vi "Create Multiline String Picture.vi"(11 "array of strings":string[](array[string])) -> (3 "string picture":picture)   [LabVIEW 2017]
doc: "Converts each string from <b>array of strings</b> into picture using custom font (Default Settings.vi:font) and places one under the other in the <b>string picture</b>."
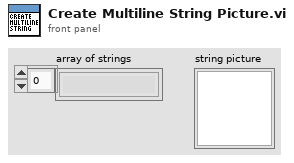
[diagram p1: front panel]
types:
  T1 = typedef "imagedata.ctl" = cluster{"image type":i32, "image depth":i32, "image":u8[], "mask":u8[], "colors":u32[], "Rectangle":cluster{"left":i16, "top":i16, "right":i16, "bottom":i16}}
  T2 = cluster{"left":i16, "top":i16, "right":i16, "bottom":i16}
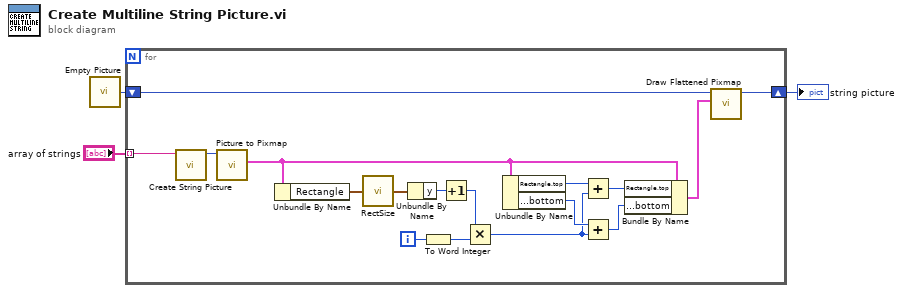
[diagram p0: block diagram]
diagram:
  n1 = call "Empty Picture"() -> ("empty picture"=w1:picture)
  n2 = for {
    shift-right: [w18] -> w2
    shift-left: w1 -> [w19]
    tunnel: "array of strings" -> [w10] mode=indexing
    i -> [w17]
    n3 = call "Create String Picture.vi"("string"=w10) -> ("string picture"=w9:picture)  [unwired: 10 in]
    n4 = call <vilib>:"Picture to Pixmap.vi"("picture"=w9) -> ("image data"=w7:T1)  [unwired: 9 in, 1 out]
    n5 = Unbundle By Name(w7) -> ("Rectangle"=w8:T2)
    n6 = call <vilib>:"RectSize.vi"("rect"=w8) -> ("point"=w6:cluster{"x":i16, "y":i16})
    n7 = Unbundle By Name(w6) -> ("y"=w4:i16)
    n8 = To Word Integer(number=w17) -> (16bit integer=w11:i16)
    n9 = Increment(x=w4) -> (x+1=w5:i16)
    n10 = Multiply(x=w5, y=w11) -> (x*y=w12:i16)
    n11 = Unbundle By Name(w7) -> ("Rectangle.top"=w16:i16, "Rectangle.bottom"=w14:i16)
    n12 = Add(x=w16, y=w12) -> (x+y=w15:i16)
    n13 = Add(x=w14, y=w12) -> (x+y=w13:i16)
    n14 = Bundle By Name(cluster=w7, "Rectangle.top"=w15, "Rectangle.bottom"=w13) -> (w20:T1)
    n15 = call <vilib>:"Draw Flattened Pixmap.vi"("image data"=w20, "picture"=w19) -> ("new picture"=w18:picture)  [unwired: 7 in]
  }
  "string picture" <- w2
